vi "MaskImage for Each Particle.vi"(8 "error in":errorcluster, 9 "Particle Variables":i32[](array[ring]) items=["Center of Mass X", "Center of Mass Y", "First Pixel X", "First Pixel Y", "Bounding Rect Left", "Bounding Rect Top", "Bounding Rect Right", "Bounding Rect Bottom", "Max Feret Diameter Start X", "Max Feret Diameter Start Y", "Max Feret Diameter End X", "Max Feret Diameter End Y", "Max Horiz. Segment Length Left", "Max Horiz. Segment Length Right", "Max Horiz. Segment Length Row", "-", "Bounding Rect Width", "Bounding Rect Height", "Bounding Rect Diagonal", "Perimeter", "Convex Hull Perimeter", "Holes' Perimeter", "Max Feret Diameter", "Equivalent Ellipse Major Axis", "Equivalent Ellipse Minor Axis", "Equivalent Ellipse Minor Axis (Feret)", "Equivalent Rect Long Side", "Equivalent Rect Short Side", "Equivalent Rect Diagonal", "Equivalent Rect Short Side (Feret)", "Average Horiz. Segment Length", "Average Vert. Segment Length", "Hydraulic Radius", "Waddel Disk Diameter", "-", "Area", "Holes' Area", "Particle & Holes' Area", "Convex Hull Area", "Image Area", "-", "Number of Holes", "Number of Horiz. Segments", "Number of Vert. Segments", "-", "Orientation", "Max Feret Diameter Orientation", "-", "% Area/Image Area", "% Area/(Particle & Holes' Area)", "Ratio of Equivalent Ellipse Axes", "Ratio of Equivalent Rect Sides", "-", "Elongation Factor", "Compactness Factor", "Heywood Circularity Factor", "Type Factor", "-", "Sum X", "Sum Y", "Sum XX", "Sum XY", "Sum YY", "Sum XXX", "Sum XXY", "Sum XYY", "Sum YYY", "-", "Moment of Inertia XX", "Moment of Inertia XY", "Moment of Inertia YY", "Moment of Inertia XXX", "Moment of Inertia XXY", "Moment of Inertia XYY", "Moment of Inertia YYY", "Norm. Moment of Inertia XX", "Norm. Moment of Inertia XY", "Norm. Moment of Inertia YY", "Norm. Moment of Inertia XXX", "Norm. Moment of Inertia XXY", "Norm. Moment of Inertia XYY", "Norm. Moment of Inertia YYY", "Hu Moment 1", "Hu Moment 2", "Hu Moment 3", "Hu Moment 4", "Hu Moment 5", "Hu Moment 6", "Hu Moment 7"], 10 "Particle Measurements (Pixels)":dbl[](array[numeric]) format="%.2f", 11 "Image":T1) -> (0 "error out":errorcluster, 3 "Image Out":T1(plugin-control))   [LabVIEW 2014]
uses:
  <vilib>/vision/Image Controls.llb/IMAQ Image.ctl
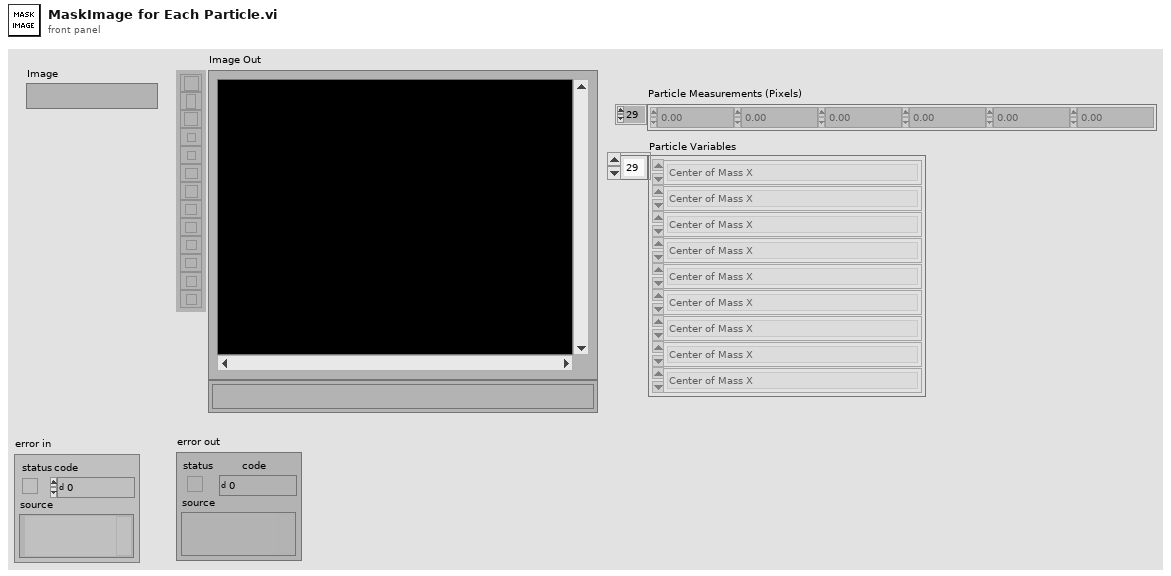
[diagram p1: front panel]
types:
  T1 = typedef "IMAQ Image.ctl" = refnum<image>
  T2 = cluster{"Global Rectangle":i32[], "Contours":cluster{"ID":enum32{"External", "Internal"}, "Type":u32, "Coordinates":i32[]}[]}
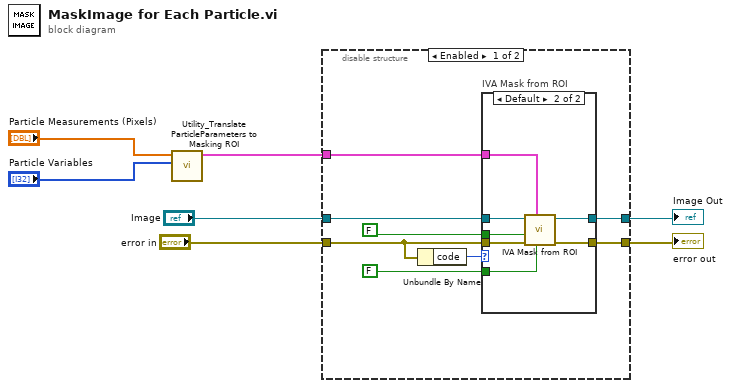
[diagram p0: block diagram]
diagram:
  n1 = call "Utility_Translate ParticleParameters to Masking ROI.vi"("Particle Variables"="Particle Variables", "Particle Measurements (Pixels)"="Particle Measurements (Pixels)") -> ("ROI Descriptor"=w3:T2)  [unwired: 9 in]
  n2 = disable-structure shown="Enabled" {
    disable-tunnel: "error in" -> [w15 w24]
    disable-tunnel: w3 -> [w14 _]
    disable-tunnel: [w12 w24] -> w6
    disable-tunnel: "Image" -> [w9 w25]
    disable-tunnel: [w8 w25] -> w5
    frame Enabled {
      n3 = Unbundle By Name(w15) -> ("code"=w10:i32)
      n4 = case "IVA Mask from ROI" shown="Default" w10 {
        tunnel: w14 -> [_ w23]
        tunnel: FALSE ("Shrink") -> [_ w22]
        tunnel: w9 -> [w16 w21]
        tunnel: w15 -> [_ w20]
        tunnel: [_ w19] -> w12
        tunnel: [w16 w18] -> w8
        tunnel: FALSE ("Out / In") -> [_ w17]
        frame -1074396199, -1074396198 {
          # "Discard\nCoordinate\nSystem\nError"
        }
        frame Default {
          n5 = call <vilib>:"IVA Mask from ROI.vi"("Shrink"=w22, "ROI Descriptor"=w23, "error in (no error)"=w20, "Out / In"=w17, "Image Src"=w21) -> ("error out"=w19:errorcluster, "Image Out"=w18:T1)  [unwired: 5 out]
        }
      }
    }
    frame Disabled {
    }
  }
  "error out" <- w6
  "Image Out" <- w5
